vi "set_position.vi"(8 "error in (no error)":errorcluster, 10 "position":i32, 11 "Bytes in":refnum<class "Bytes.lvclass">) -> (0 "error out":errorcluster, 3 "Bytes out":refnum<class "Bytes.lvclass">)   [LabVIEW 2020, in "Bytes.lvclass"]
uses:
  Bytes.lvclass
  Bytes.lvclass/Bytes.ctl
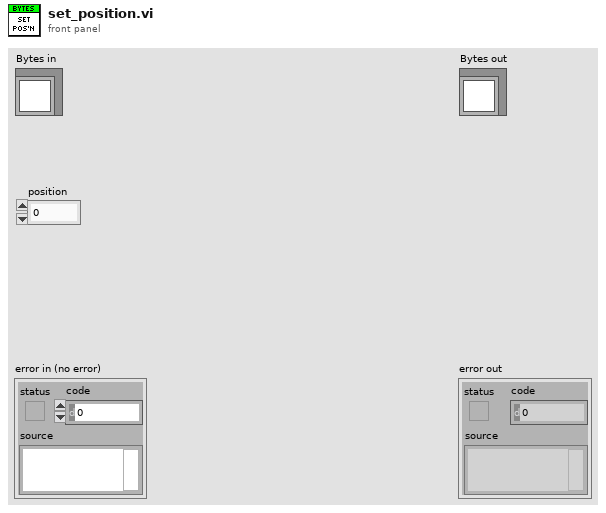
[diagram p1: front panel]
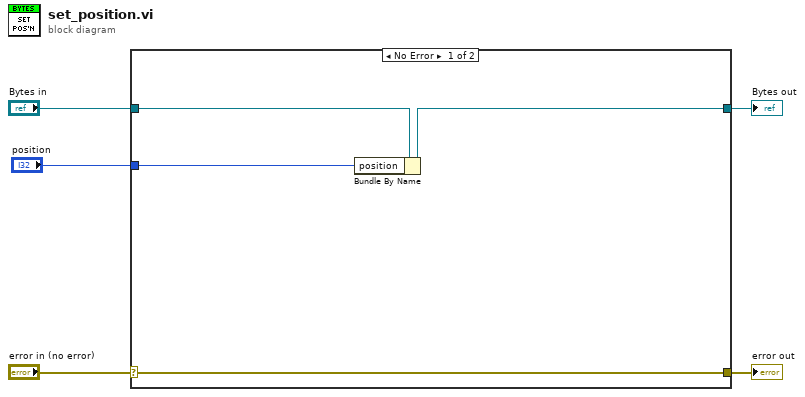
[diagram p0: block diagram]
diagram:
  n1 = case shown="No Error" "error in (no error)" {
    selector: "error in (no error)" -> [w8 w11]
    tunnel: [w8 w11] -> w4
    tunnel: [w7 w10] -> w2
    tunnel: "Bytes in" -> [w9 w10]
    tunnel: "position" -> [w6 _]
    frame No Error {
      n2 = Bundle By Name(cluster=w9, "position"=w6) -> (w7:refnum<class "Bytes.lvclass">)
    }
    frame Error {
    }
  }
  "error out" <- w4
  "Bytes out" <- w2
